vi "Baseline_remove.vi"(9 "B array":dbl[](array[numeric]), 10 "Averaged I(B) In":dbl[][](array[numeric]), 11 "B0":dbl) -> (2 "Array":dbl[][](array[numeric]), 3 "BaselineSubtracted I(B)":dbl[][](array[numeric]))   [LabVIEW 2015]
uses:
  <vilib>/Analysis/baseanly.llb/Mean (DBL).vi
  <vilib>/Analysis/NI_AALBase.lvlib
panel:
  out "I(B) out":T1(graph)
  out "mean 2":dbl format="%0.2f"
  out "mean 1":dbl format="%0.2f"
  out "Ending":T1(graph)
  out "I(B) in":T1(graph)
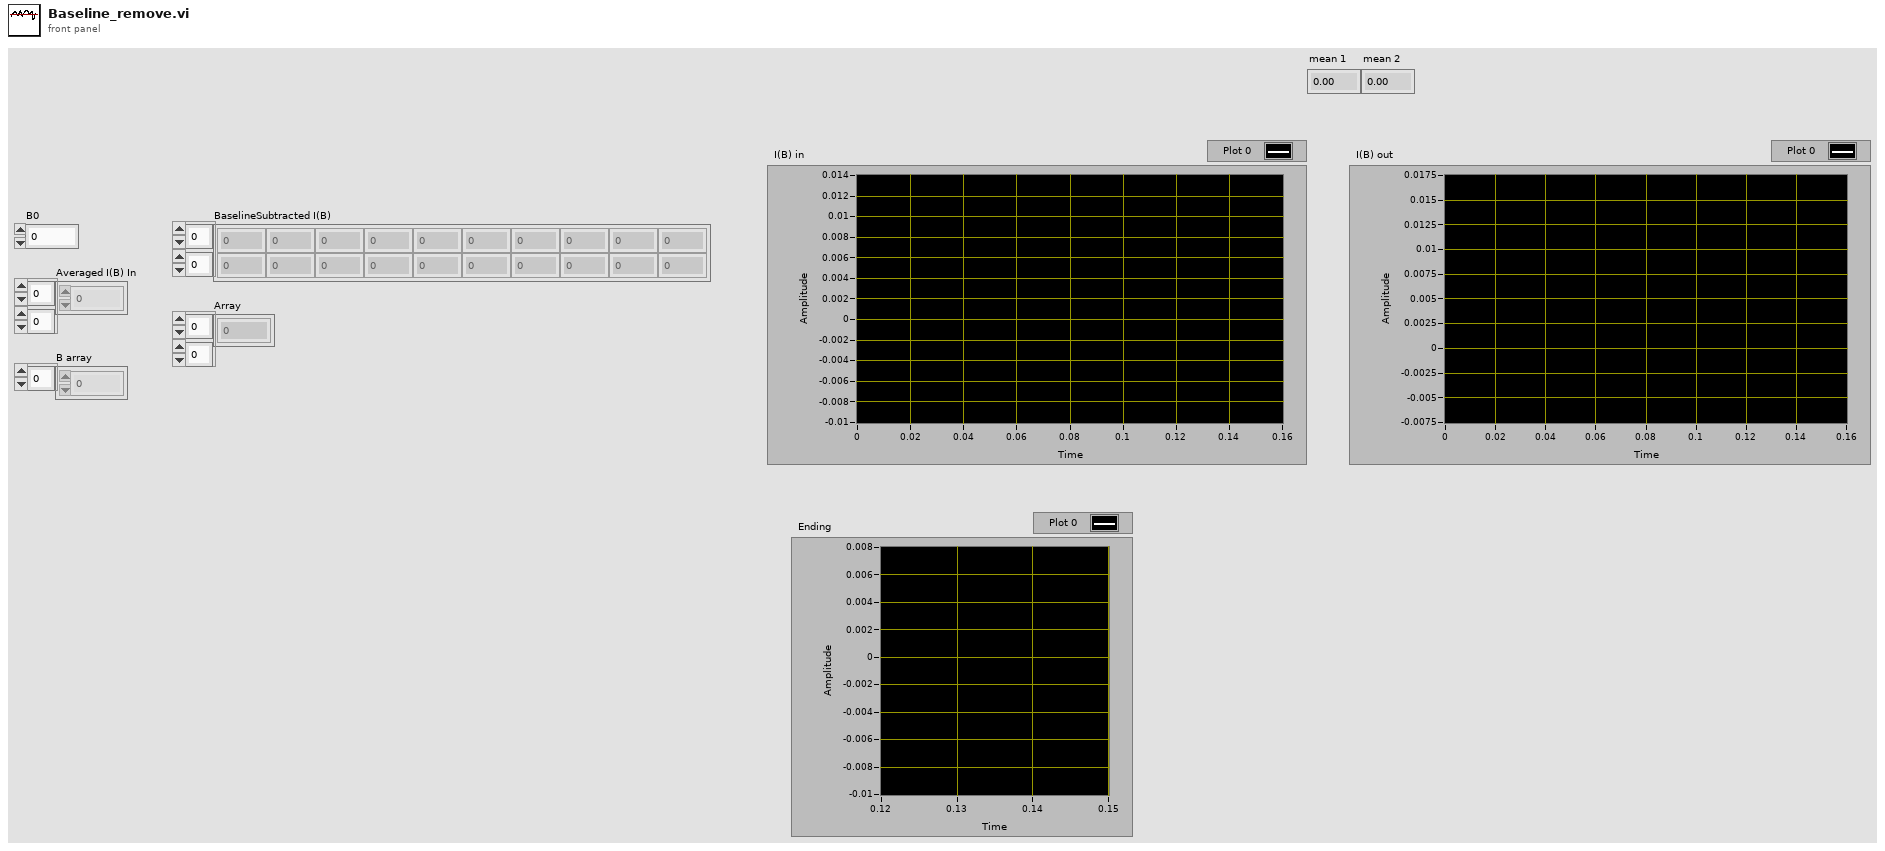
[diagram p1: front panel]
types:
  T1 = cluster{"B array":dbl[], "Averaged I(B) In":dbl[]}[]
  T2 = cluster{"B array":dbl[], "Averaged I(B) In":dbl[]}
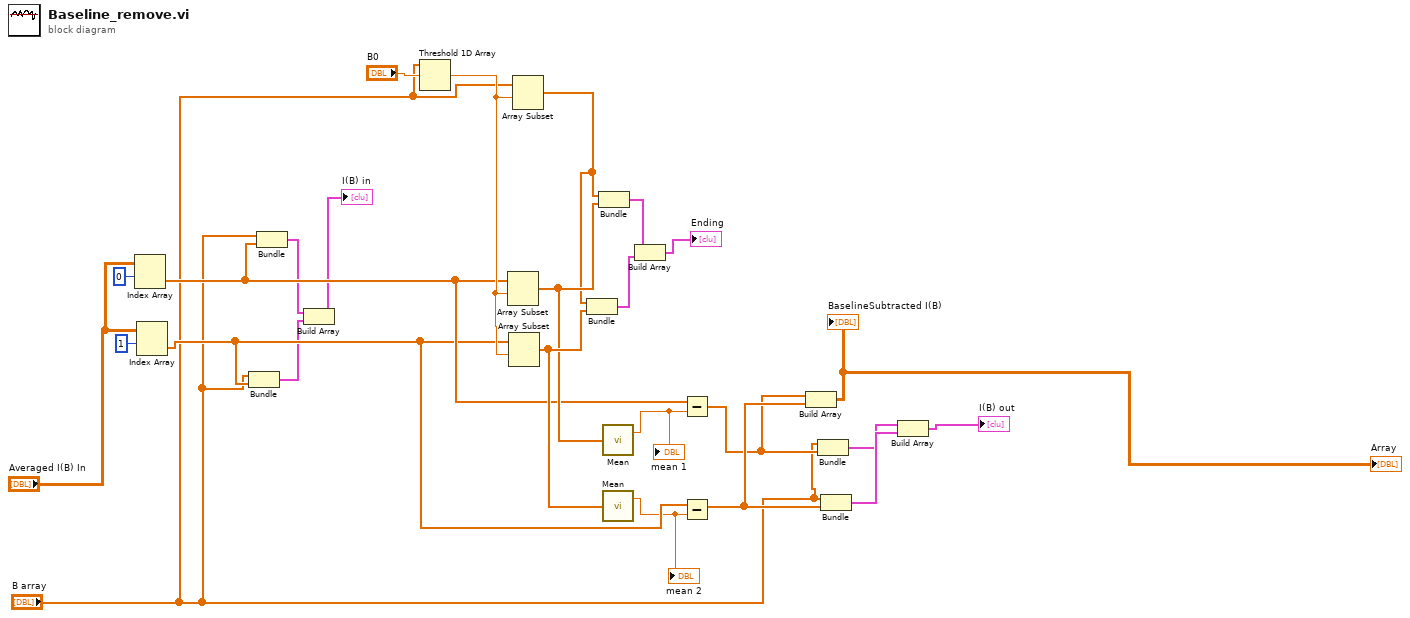
[diagram p0: block diagram]
diagram:
  n1 = Index Array(array="Averaged I(B) In", index (row)=0) -> (element=w9:dbl[])  [unwired: 1 in]
  n2 = Index Array(array="Averaged I(B) In", index (row)=1) -> (element=w8:dbl[])  [unwired: 1 in]
  n3 = Bundle("B array"="B array", "Averaged I(B) In"=w8) -> (w7:T2)  [unwired: 1 in]
  n4 = Bundle("B array"="B array", "Averaged I(B) In"=w9) -> (w6:T2)  [unwired: 1 in]
  n5 = Build Array(w6, w7) -> (→"I(B) in":T1)
  n6 = Threshold 1D Array(2:"B0", 3:"B array") -> (0:w13:dbl)  [unwired: 1 in]
  n7 = Array Subset(array=w9, index=w13) -> (w17:dbl[])  [unwired: 1 in]
  n8 = Array Subset(array=w8, index=w13) -> (w18:dbl[])  [unwired: 1 in]
  n9 = Array Subset(array="B array", index=w13) -> (w14:dbl[])  [unwired: 1 in]
  n10 = Bundle(w14, w18) -> (w16:cluster{dbl[], dbl[]})  [unwired: 1 in]
  n11 = Bundle(w14, w17) -> (w15:cluster{dbl[], dbl[]})  [unwired: 1 in]
  n12 = call-poly <vilib>:"Mean.vi"("X"=w17) -> ("mean"=w19:dbl)  [unwired: 1 out]
  "mean 1" <- w19
  n13 = call-poly <vilib>:"Mean.vi"("X"=w18) -> ("mean"=w3:dbl)  [unwired: 1 out]
  "mean 2" <- w3
  n14 = Build Array(w15, w16) -> (→"Ending":cluster{dbl[], dbl[]}[])
  n15 = Subtract(x=w9, y=w19) -> (x-y=w23:dbl[])
  n16 = Subtract(x=w8, y=w3) -> (x-y=w24:dbl[])
  n17 = Build Array(w23, w24) -> (→"BaselineSubtracted I(B)" →"Array":dbl[][])
  n18 = Bundle("B array"="B array", w23) -> (w20:cluster{"B array":dbl[], dbl[]})  [unwired: 1 in]
  n19 = Bundle("B array"="B array", w24) -> (w21:cluster{"B array":dbl[], dbl[]})  [unwired: 1 in]
  n20 = Build Array(w20, w21) -> (→"I(B) out":cluster{"B array":dbl[], dbl[]}[])
